vi "RSZVB Select Power Meter.vi"(6 "Power Meter (1)":i32=1, 7 "Out Port (1)":i32=1, 8 "error in (no error)":errorcluster {"code" format="%.0x"}, 9 "Trace Name (Trc1)":string="Trc1", 10 "Channel (1)":i32=1, 11 "VISA session":refnum<visa-resource-name>) -> (0 "error out":errorcluster {"code" format="%.0x"}, 3 "dup VISA session":refnum<visa-resource-name>)   [LabVIEW 2011]
doc: "This VI selects one of two powermeters for the given drive ports into the given trace to prepare a power calibration.\n\nRemote-control command(s):\nCALCulate<Ch>:PARameter:SDEFine '<string>', 'Pmtr1D1' | ...\nCALCulate<Ch>:PARameter:MEASure '<string>', 'Pmtr1D1' | ..."
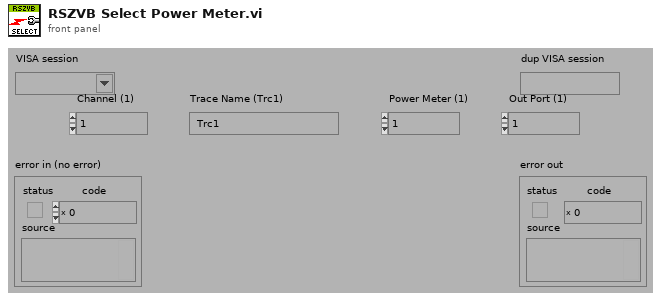
[diagram p1: front panel]
types:
  T1 = cluster{"Error Checking (T: On)":bool, "Installed Options":string[], "Data Valid?":bool, "Ports":i32, "Model":string[], "Option Checking (T: On)":bool}
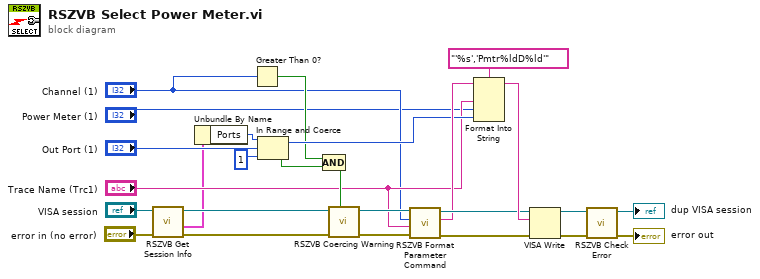
[diagram p0: block diagram]
diagram:
  n1 = call "RSZVB Get Session Info.vi"("error in (no error)"="error in (no error)", "VISA session"="VISA session") -> ("error out"=w5:errorcluster, "Session Info"=w3:T1, "dup VISA session"=w4:refnum<visa-resource-name>)  [unwired: 7 in]
  n2 = Unbundle By Name(w3) -> ("Ports"=w2:i32)
  n3 = Greater Than 0?(x="Channel (1)") -> (x > 0?=w15:bool)
  n4 = In Range and Coerce(upper limit=w2, x="Out Port (1)", lower limit=1) -> (coerced(x)=w16:i32, In Range?=w14:bool)
  n5 = Compound Arithmetic op=AND(w15, w14) -> (w23:bool)
  n6 = call "RSZVB Coercing Warning.vi"("In Range?"=w23, "error in (no error)"=w5, "VISA session"=w4) -> ("error out"=w20:errorcluster, "dup VISA session"=w19:refnum<visa-resource-name>)  [unwired: 7 in]
  n7 = call "RSZVB Format Parameter Command.vi"("error in (no error)"=w20, "Trace Name (Trc1)"="Trace Name (Trc1)", "Channel (1)"="Channel (1)", "VISA session"=w19) -> ("error out"=w21:errorcluster, "Buffer"=w17:string, "dup VISA session"=w18:refnum<visa-resource-name>)  [unwired: 5 in]
  n8 = Format Into String(format string="'%s','Pmtr%ldD%ld'", initial string=w17, "Trace Name (Trc1)", "Power Meter (1)", w16) -> (resulting string=w22:string)  [unwired: 1 in, 1 out]
  n9 = VISA Write(VISA resource name=w18, write buffer=w22, error in (no error)=w21) -> (VISA resource name out=w24:refnum<visa-resource-name>, error out=w25:errorcluster)  [unwired: 1 out]
  n10 = call "RSZVB Check Error.vi"("error in (no error)"=w25, "VISA session"=w24) -> ("error out"=→"error out":errorcluster, "dup VISA session"=→"dup VISA session":refnum<visa-resource-name>)  [unwired: 8 in]
